vi "Create RC Server.vi"(8 "error in (no error)":errorcluster, 11 "RemoteControl in":refnum<class "RemoteControl.lvclass">) -> (0 "error out":errorcluster, 3 "RemoteControl out":refnum<class "RemoteControl.lvclass">)   [LabVIEW 2019, in "RemoteControl.lvclass"]
uses:
  RemoteControl.lvclass
  Typedefs/RC Process Type--Enum.ctl
  RemoteControl.lvclass/RemoteControl.ctl
  <vilib>/JKI/JKI SMO/SMO/Typedefs/Public Events.ctl
  <vilib>/JKI/JKI SMO/SMO/Typedefs/SMOState --Enum.ctl
  <vilib>/JKI/JKI SMO/SMO/Typedefs/Reserve State--Enum.ctl
  Typedefs/PublicEvents--Cluster.ctl
  Typedefs/PublicEvents--RemoteControl.SendMessageFromProcess.ctl
  Typedefs/Message--Cluster.ctl
  <vilib>/JKI/JKI SMO/SMO/SMO.lvclass
  C:/Program Files (x86)/National Instruments/LabVIEW 2019/vi.lib/JKI/JKI SMO/SMO/SMO.lvclass
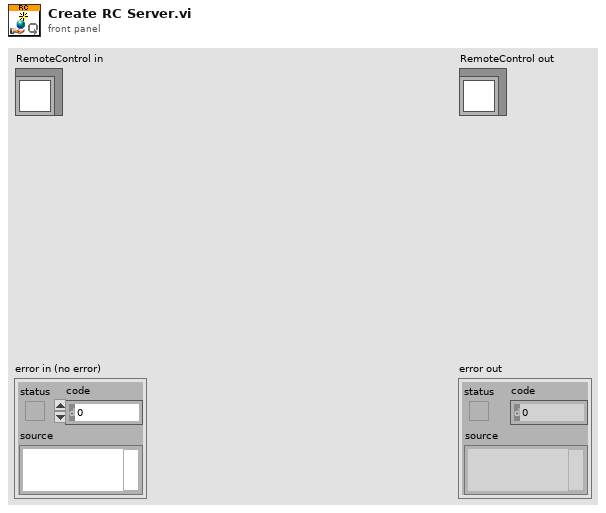
[diagram p1: front panel]
types:
  T1 = typedef "RemoteControl.lvclass/RC Process Type--Enum.ctl" = enum16{"Connection Monitor", "Server", "Client"}
  T2 = typedef "RemoteControl.lvclass/PublicEvents--Cluster.ctl" = cluster{"SendMessageFromProcess":refnum<user-event>}
  T3 = typedef "SMO.lvclass/Public Events.ctl" = cluster{"Error":refnum<user-event>, "State":refnum<user-event>, "Reserve State":refnum<user-event>}
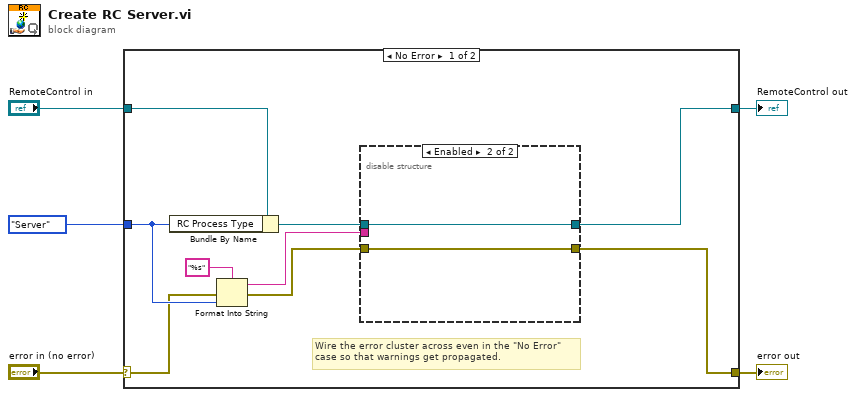
[diagram p0: block diagram]
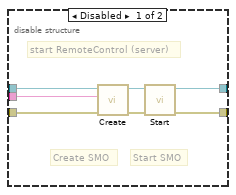
[diagram p2: hidden frame]
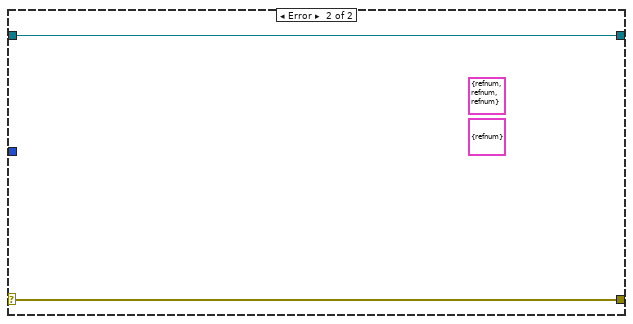
[diagram p3: hidden frame]
diagram:
  n1 = case shown="No Error" "error in (no error)" {
    selector: "error in (no error)" -> [w7 w25]
    tunnel: [w12 w25] -> w4
    tunnel: [w11 w24] -> w2
    tunnel: "RemoteControl in" -> [w13 w24]
    tunnel: RC_Process_Type--Enum."Server" ("RC Process Type") -> [w9 _]
    frame No Error {
      # "Wire the error cluster across even in the \"No Error\"\ncase so that warnings get propagated."
      n2 = Bundle By Name(cluster=w13, "RC Process Type"=w9) -> (w14:refnum<class "RemoteControl.lvclass">)
      n3 = Format Into String(format string="%s", error in=w7, w9) -> (resulting string=w8:string, error out=w6:errorcluster)  [unwired: 1 in]
      n4 = disable-structure shown="Enabled" {
        disable-tunnel: w14 -> [w19 w22]
        disable-tunnel: [w18 w23] -> w12
        disable-tunnel: [w17 w22] -> w11
        disable-tunnel: w8 -> [w16 _]
        disable-tunnel: w6 -> [w15 w23]
        frame Disabled {
          # "start RemoteControl (server)"
          # "Start SMO"
          # "Create SMO"
          n5 = call <vilib>:"Create.vi"("error in (no error)"=w15, "Subsystem Name (optional)"=w16, "SMO"=w19) -> ("error out"=w21:errorcluster, "SMO out"=w20:refnum<class "RemoteControl.lvclass">)  [unwired: 6 in, 1 out]
          n6 = call <vilib>:"Start.vi"("error in (no error)"=w21, "SMO"=w20) -> ("error out"=w18:errorcluster, "SMO out"=w17:refnum<class "RemoteControl.lvclass">)  [unwired: 8 in]
        }
        frame Enabled {
        }
      }
    }
    frame Error {
      (unwired) T2 {"SendMessageFromProcess"=refnum} ("RC Public Events")
      (unwired) T3 {"Error"=refnum, "State"=refnum, "Reserve State"=refnum} ("Public Events")
    }
  }
  "error out" <- w4
  "RemoteControl out" <- w2
